vi "Auto1Tote.vi"(8 "error in":errorcluster) -> ()   [LabVIEW 2014]
uses:
  <vilib>/Rock Robotics/WPI/DriverStation/WPI_DriverStationRobotMode2.ctl
  LowerLiftAndOpenArms.ctl
  Robot Global Data.vi
  Gantry/GantryGlobals.vi
  AutomationGlobals.vi
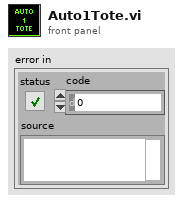
[diagram p1: front panel]
types:
  T1 = enum16{"WaitForInput", "GantryOut", "Lift", "Forward", "Autostack", "Left", "PutToteDown", "GrabBarrelLift", "Right", "Forward2", "Done"}
  T2 = typedef "WPI_DriverStationRobotMode2.ctl" = enum16{"Autonomous Disabled", "Autonomous Enabled", "Teleop Disabled", "Teleop Enabled", "Disconnected", "Finish", "Test Disabled", "Test Enabled", "Emergency Stopped"}
  T3 = typedef "LowerLiftAndOpenArms.ctl" = enum16{"WaitingForInput", "LowerLift", "OpenArms", "LowerLiftMore", "CloseArms", "RaiseLift", "StopArms"}
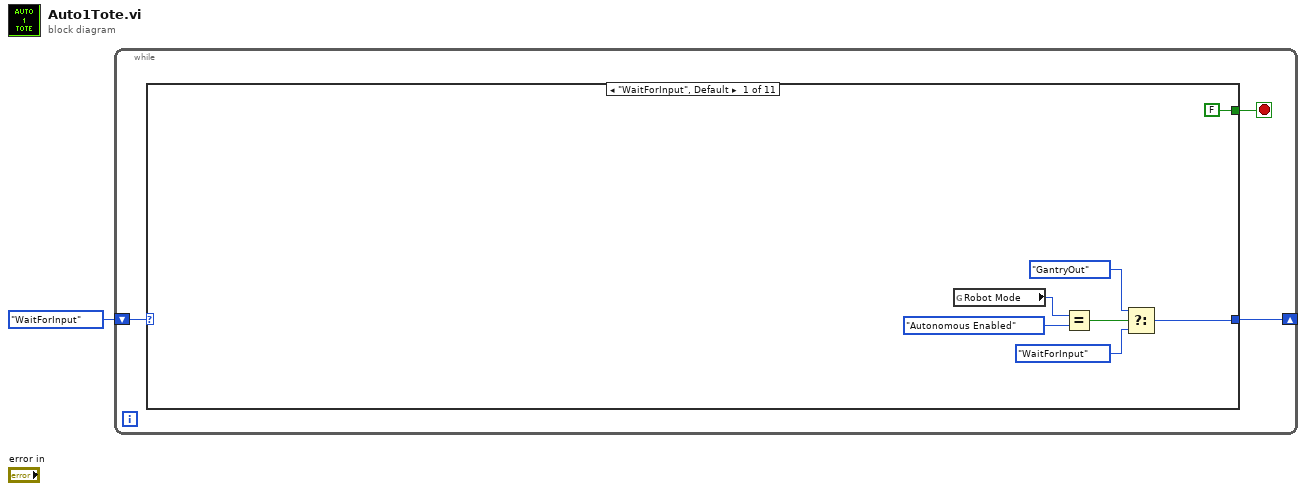
[diagram p0: block diagram]
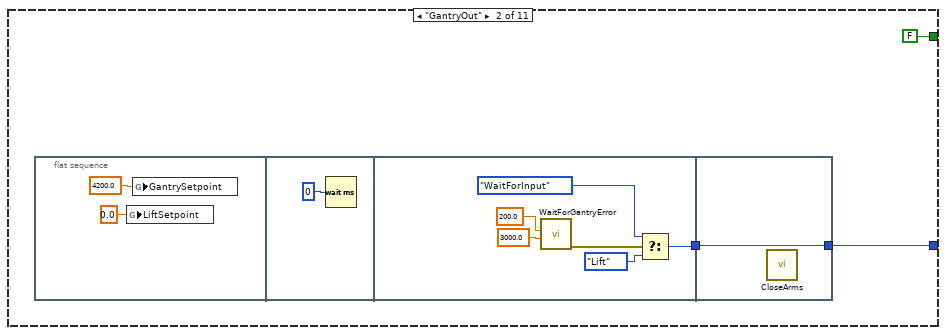
[diagram p2: hidden frame]
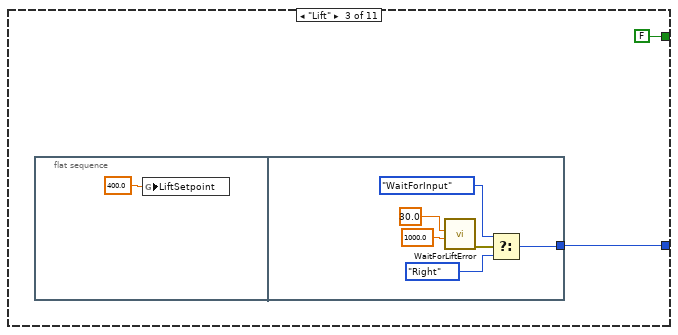
[diagram p3: hidden frame]
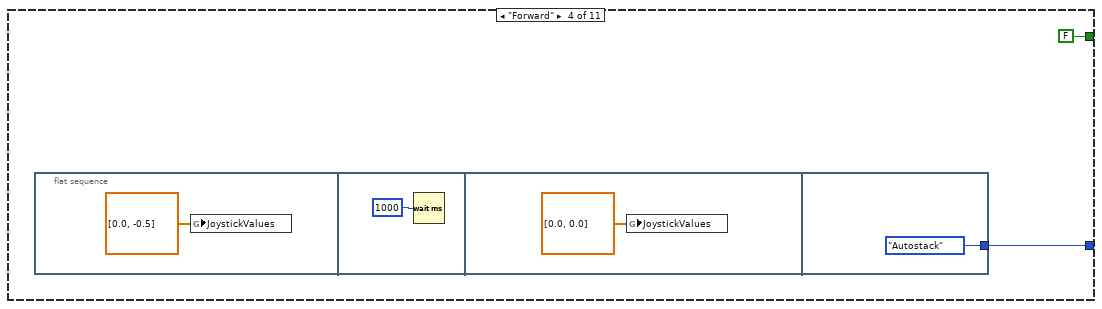
[diagram p4: hidden frame]
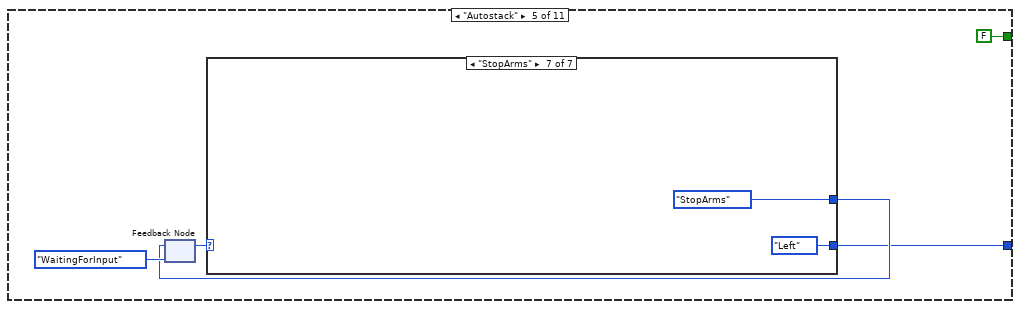
[diagram p5: hidden frame]
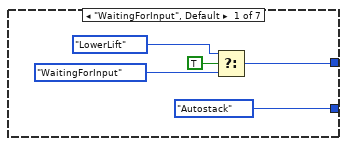
[diagram p6: hidden frame]
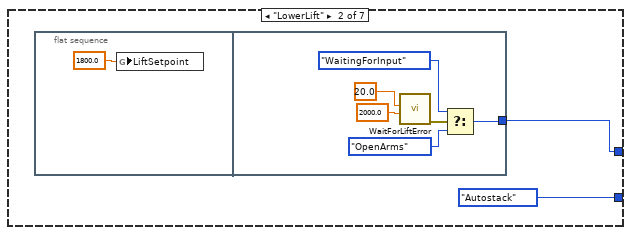
[diagram p7: hidden frame]
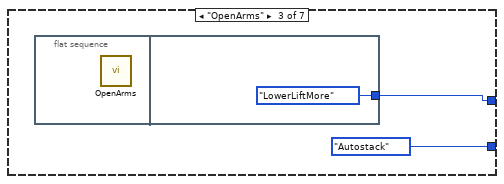
[diagram p8: hidden frame]
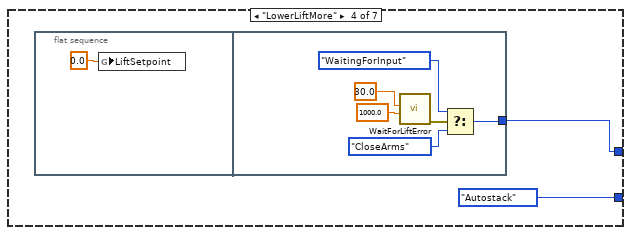
[diagram p9: hidden frame]
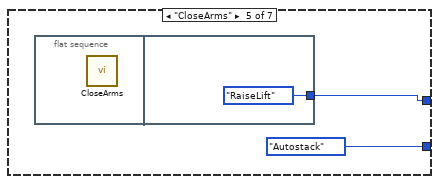
[diagram p10: hidden frame]
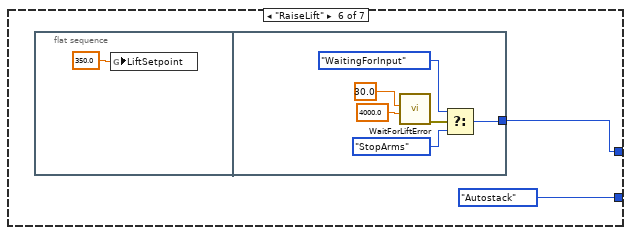
[diagram p11: hidden frame]
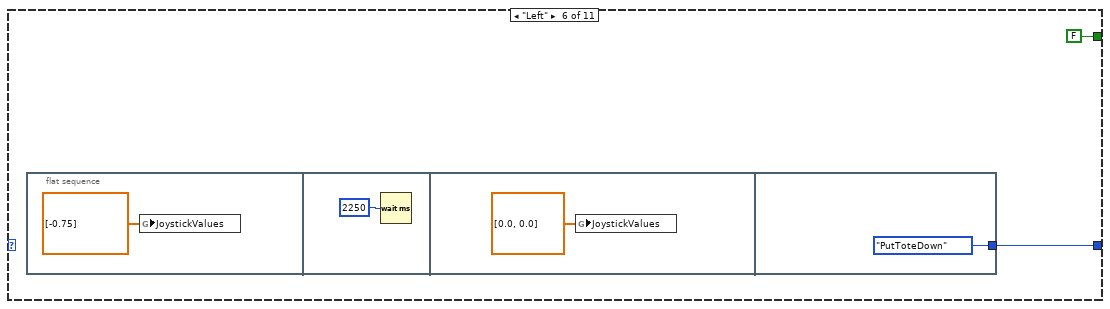
[diagram p12: hidden frame]
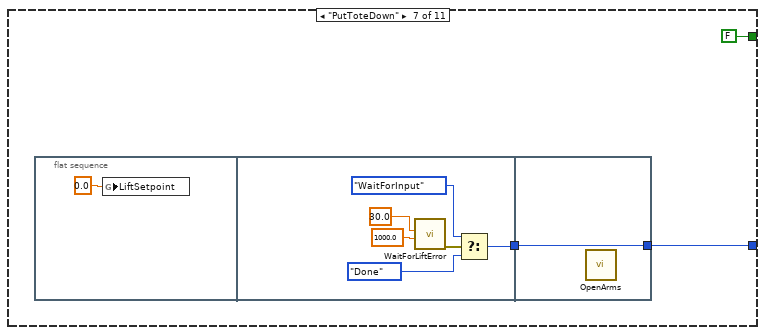
[diagram p13: hidden frame]
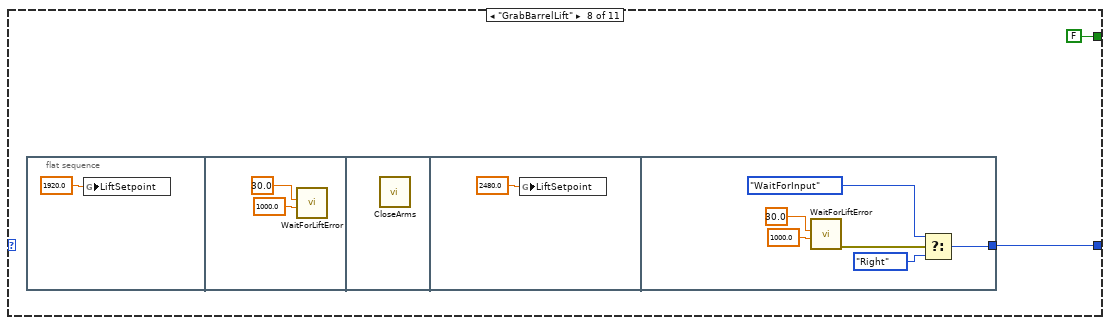
[diagram p14: hidden frame]
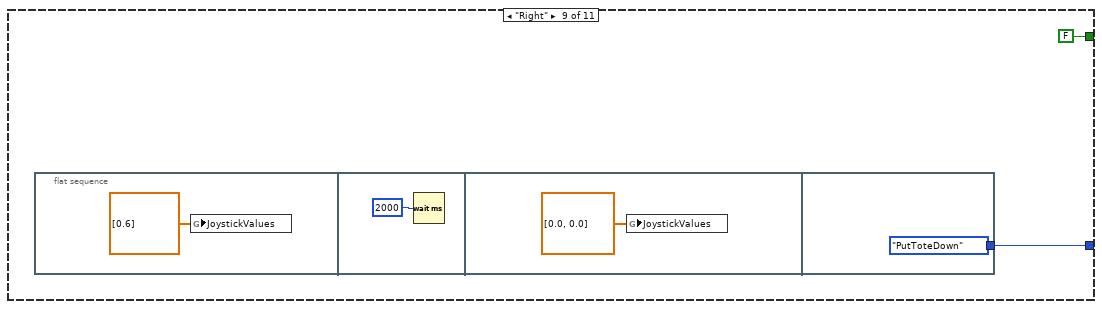
[diagram p15: hidden frame]
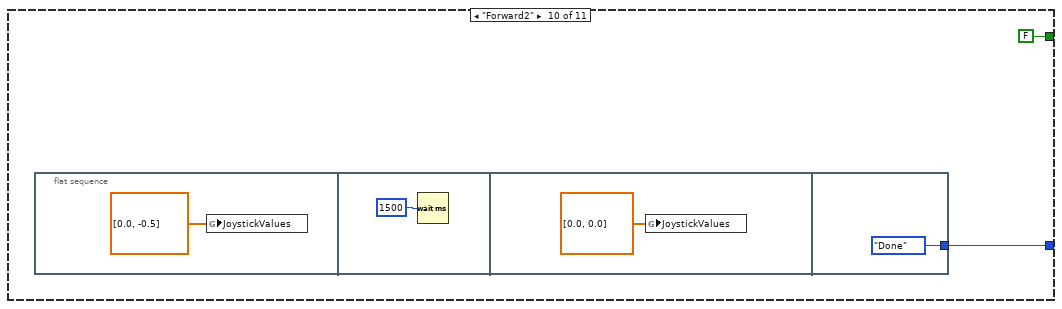
[diagram p16: hidden frame]
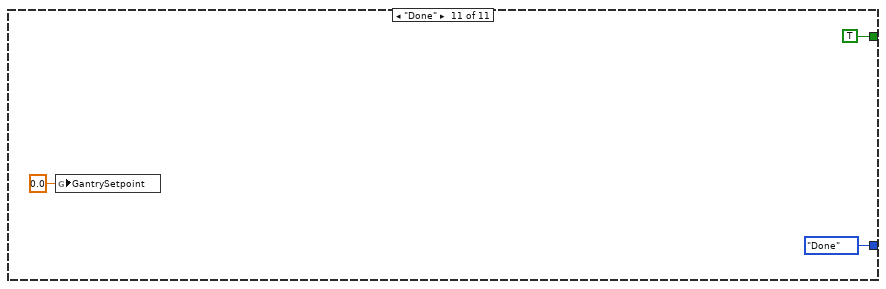
[diagram p17: hidden frame]
diagram:
  n1 = while {
    shift-right: [w3] -> _
    shift-left: T1."WaitForInput" ("Enum") -> [w4]
    stop <- w2 stop-if-true
    n2 = case shown="\"WaitForInput\", Default" w4 {
      tunnel: [w8 w14 w26 w34 w40 w85 w92 w102 w114 w121 T1."Done" ("Enum")] -> w3
      tunnel: [FALSE FALSE FALSE FALSE FALSE FALSE FALSE FALSE FALSE FALSE TRUE] -> w2
      frame "WaitForInput", Default {
        n3 = global read "Robot Global Data.vi" "Robot Mode"() -> (w11:T2)
        n4 = Equal?(x=w11, y=WPI_DriverStationRobotMode2."Autonomous Enabled") -> (x = y?=w9:bool)
        n5 = Select(t=T1."GantryOut" ("Enum"), s=w9, f=T1."WaitForInput" ("Enum")) -> (s? t:f=w8:T1)
      }
      frame "GantryOut" {
        n6 = flat-sequence {
          tunnel: [w20] -> w12
          tunnel: [w24] -> w14
          tunnel: w12 -> [w24]
          frame #0 {
            n7 = global write "GantryGlobals.vi" "LiftSetpoint"(0.0 ("LiftSetpoint")) -> ()
            n8 = global write "GantryGlobals.vi" "GantrySetpoint"(4200.0 ("GantrySetpoint")) -> ()
          }
          frame #1 {
            n9 = Wait (ms)(milliseconds to wait=u32 0) -> ()  [unwired: 1 out]
          }
          frame #2 {
            n10 = call "WaitForGantryError.vi"("Timeout (ms)"=3000.0, "AllowedError"=200.0) -> ("error out"=w21:errorcluster)  [unwired: 9 in]
            n11 = Select(t=T1."WaitForInput" ("Enum"), s=w21, f=T1."Lift" ("Enum")) -> (s? t:f=w20:T1)
          }
          frame #3 {
            n12 = call "CloseArms.vi"() -> ()  [unwired: 12 in]
          }
        }
      }
      frame "Lift" {
        n13 = flat-sequence {
          tunnel: [w30] -> w26
          frame #0 {
            n14 = global write "GantryGlobals.vi" "LiftSetpoint"(400.0 ("LiftSetpoint")) -> ()
          }
          frame #1 {
            n15 = call "WaitForLiftError.vi"("Timeout (ms)"=1000.0, "AllowedError"=30.0) -> ("error out"=w33:errorcluster)  [unwired: 9 in]
            n16 = Select(t=T1."WaitForInput" ("Enum"), s=w33, f=T1."Right" ("Enum")) -> (s? t:f=w30:T1)
          }
        }
      }
      frame "Forward" {
        n17 = flat-sequence {
          tunnel: [T1."Autostack" ("Enum")] -> w34
          frame #0 {
            n18 = global write "AutomationGlobals.vi" "JoystickValues"(dbl[] [0.0, -0.5] ("s? t:f")) -> ()
          }
          frame #1 {
            n19 = Wait (ms)(milliseconds to wait=u32 1000) -> ()  [unwired: 1 out]
          }
          frame #2 {
            n20 = global write "AutomationGlobals.vi" "JoystickValues"(dbl[] [0.0, 0.0] ("s? t:f")) -> ()
          }
          frame #3 {
          }
        }
      }
      frame "Autostack" {
        n21 = feedback #1(LowerLiftAndOpenArms."WaitingForInput" ("LowerAndOpen")) -> (w42:T3)
        n22 = case shown="\"StopArms\"" w42 {
          tunnel: [w47 w51 w60 w63 w72 w75 LowerLiftAndOpenArms."StopArms" ("LowerAndOpen")] -> w41
          tunnel: [T1."Autostack" ("Enum") T1."Autostack" ("Enum") T1."Autostack" ("Enum") T1."Autostack" ("Enum") T1."Autostack" ("Enum") T1."Autostack" ("Enum") T1."Left" ("Enum")] -> w40
          frame "WaitingForInput", Default {
            n23 = Select(t=LowerLiftAndOpenArms."LowerLift" ("LowerAndOpen"), s=TRUE, f=LowerLiftAndOpenArms."WaitingForInput" ("LowerAndOpen")) -> (s? t:f=w47:T3)
          }
          frame "LowerLift" {
            n24 = flat-sequence {
              tunnel: [w53] -> w51
              frame #0 {
                n25 = global write "GantryGlobals.vi" "LiftSetpoint"(1800.0 ("LiftSetpoint")) -> ()
              }
              frame #1 {
                n26 = call "WaitForLiftError.vi"("Timeout (ms)"=2000.0, "AllowedError"=20.0) -> ("error out"=w56:errorcluster)  [unwired: 9 in]
                n27 = Select(t=LowerLiftAndOpenArms."WaitingForInput" ("LowerAndOpen"), s=w56, f=LowerLiftAndOpenArms."OpenArms" ("LowerAndOpen")) -> (s? t:f=w53:T3)
              }
            }
          }
          frame "OpenArms" {
            n28 = flat-sequence {
              tunnel: [LowerLiftAndOpenArms."LowerLiftMore" ("LowerAndOpen")] -> w60
              frame #0 {
                n29 = call "OpenArms.vi"() -> ()  [unwired: 12 in]
              }
              frame #1 {
              }
            }
          }
          frame "LowerLiftMore" {
            n30 = flat-sequence {
              tunnel: [w65] -> w63
              frame #0 {
                n31 = global write "GantryGlobals.vi" "LiftSetpoint"(0.0 ("LiftSetpoint")) -> ()
              }
              frame #1 {
                n32 = call "WaitForLiftError.vi"("Timeout (ms)"=1000.0, "AllowedError"=30.0) -> ("error out"=w68:errorcluster)  [unwired: 9 in]
                n33 = Select(t=LowerLiftAndOpenArms."WaitingForInput" ("LowerAndOpen"), s=w68, f=LowerLiftAndOpenArms."CloseArms" ("LowerAndOpen")) -> (s? t:f=w65:T3)
              }
            }
          }
          frame "CloseArms" {
            n34 = flat-sequence {
              tunnel: [LowerLiftAndOpenArms."RaiseLift" ("LowerAndOpen")] -> w72
              frame #0 {
                n35 = call "CloseArms.vi"() -> ()  [unwired: 12 in]
              }
              frame #1 {
              }
            }
          }
          frame "RaiseLift" {
            n36 = flat-sequence {
              tunnel: [w77] -> w75
              frame #0 {
                n37 = global write "GantryGlobals.vi" "LiftSetpoint"(350.0 ("LiftSetpoint")) -> ()
              }
              frame #1 {
                n38 = call "WaitForLiftError.vi"("Timeout (ms)"=4000.0, "AllowedError"=30.0) -> ("error out"=w80:errorcluster)  [unwired: 9 in]
                n39 = Select(t=LowerLiftAndOpenArms."WaitingForInput" ("LowerAndOpen"), s=w80, f=LowerLiftAndOpenArms."StopArms" ("LowerAndOpen")) -> (s? t:f=w77:T3)
              }
            }
          }
          frame "StopArms" {
          }
        }
        n40 = feedback-in #1(w41) -> ()
      }
      frame "Left" {
        n41 = flat-sequence {
          tunnel: [T1."PutToteDown" ("Enum")] -> w85
          frame #0 {
            n42 = global write "AutomationGlobals.vi" "JoystickValues"(dbl[] [-0.75] ("s? t:f")) -> ()
          }
          frame #1 {
            n43 = Wait (ms)(milliseconds to wait=u32 2250) -> ()  [unwired: 1 out]
          }
          frame #2 {
            n44 = global write "AutomationGlobals.vi" "JoystickValues"(dbl[] [0.0, 0.0] ("s? t:f")) -> ()
          }
          frame #3 {
          }
        }
      }
      frame "PutToteDown" {
        n45 = flat-sequence {
          tunnel: [w97] -> w91
          tunnel: [w101] -> w92
          tunnel: w91 -> [w101]
          frame #0 {
            n46 = global write "GantryGlobals.vi" "LiftSetpoint"(0.0 ("LiftSetpoint")) -> ()
          }
          frame #1 {
            n47 = call "WaitForLiftError.vi"("Timeout (ms)"=1000.0, "AllowedError"=30.0) -> ("error out"=w100:errorcluster)  [unwired: 9 in]
            n48 = Select(t=T1."WaitForInput" ("Enum"), s=w100, f=T1."Done" ("Enum")) -> (s? t:f=w97:T1)
          }
          frame #2 {
            n49 = call "OpenArms.vi"() -> ()  [unwired: 12 in]
          }
        }
      }
      frame "GrabBarrelLift" {
        n50 = flat-sequence {
          tunnel: [w113] -> w102
          frame #0 {
            n51 = global write "GantryGlobals.vi" "LiftSetpoint"(1920.0 ("LiftSetpoint")) -> ()
          }
          frame #1 {
            n52 = call "WaitForLiftError.vi"("Timeout (ms)"=1000.0, "AllowedError"=30.0) -> ()  [unwired: 9 in, 1 out]
          }
          frame #2 {
            n53 = call "CloseArms.vi"() -> ()  [unwired: 12 in]
          }
          frame #3 {
            n54 = global write "GantryGlobals.vi" "LiftSetpoint"(2480.0 ("LiftSetpoint")) -> ()
          }
          frame #4 {
            n55 = call "WaitForLiftError.vi"("Timeout (ms)"=1000.0, "AllowedError"=30.0) -> ("error out"=w112:errorcluster)  [unwired: 9 in]
            n56 = Select(t=T1."WaitForInput" ("Enum"), s=w112, f=T1."Right" ("Enum")) -> (s? t:f=w113:T1)
          }
        }
      }
      frame "Right" {
        n57 = flat-sequence {
          tunnel: [T1."PutToteDown" ("Enum")] -> w114
          frame #0 {
            n58 = global write "AutomationGlobals.vi" "JoystickValues"(dbl[] [0.6] ("s? t:f")) -> ()
          }
          frame #1 {
            n59 = Wait (ms)(milliseconds to wait=u32 2000) -> ()  [unwired: 1 out]
          }
          frame #2 {
            n60 = global write "AutomationGlobals.vi" "JoystickValues"(dbl[] [0.0, 0.0] ("s? t:f")) -> ()
          }
          frame #3 {
          }
        }
      }
      frame "Forward2" {
        n61 = flat-sequence {
          tunnel: [T1."Done" ("Enum")] -> w121
          frame #0 {
            n62 = global write "AutomationGlobals.vi" "JoystickValues"(dbl[] [0.0, -0.5] ("s? t:f")) -> ()
          }
          frame #1 {
            n63 = Wait (ms)(milliseconds to wait=u32 1500) -> ()  [unwired: 1 out]
          }
          frame #2 {
            n64 = global write "AutomationGlobals.vi" "JoystickValues"(dbl[] [0.0, 0.0] ("s? t:f")) -> ()
          }
          frame #3 {
          }
        }
      }
      frame "Done" {
        n65 = global write "GantryGlobals.vi" "GantrySetpoint"(0.0 ("GantrySetpoint")) -> ()
      }
    }
  }
